vi "fil1_calc.vi"(6 "Detector 3 Correlation In":i32, 7 "Detector 1 Correlation In":i32, 8 "AI1":i32, 9 "AI0":i32) -> (1 "Detector 3 Correlation Out":i32, 3 "Detector 1 Correlation Out":i32)   [LabVIEW 2012]
uses:
  <vilib>/rvi/Emulation/niFpgaSctlEmulationGetInTimedLoop.vi
  <vilib>/rvi/DataTransferAndStorage/Container/Common/niFpgaContainerGetUniqueNameForEmu.vi
  <vilib>/rvi/FIFO/Fifo_Resource/nirvififoEmulationSetSize.vi
  <vilib>/rvi/errors/niFpgaSetErrorForExecOnDevCompSimple.vi
  <vilib>/rvi/eio/common/nirviEmuReportErrorAndStop.vi
  <vilib>/rvi/Emulation/niFpgaSctlEmulationFifoFullMgr.vi
  <vilib>/rvi/Emulation/niFpgaSctlEmulationResourceMgr.vi
  <vilib>/rvi/DataTransferAndStorage/Container/XNode/niFpgaContainer.xnode
  <vilib>/rvi/FIFO/Fifo_Resource/nirvififoEmulationWrite.vi
  <vilib>/rvi/FIFO/Fifo_Resource/nirvififoEmulationRead.vi
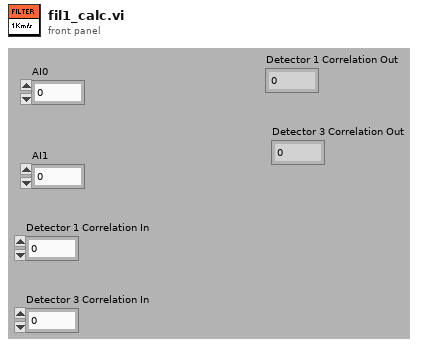
[diagram p1: front panel]
types:
  T1 = cluster{"Average Out":i32, "Next State":u16, "Detector 1 Correlation out":i32, "Detector 3 Correlation out":i32, "Velocity Count out":i32, "Detector counter out":i32, "Timeout count out":u32}
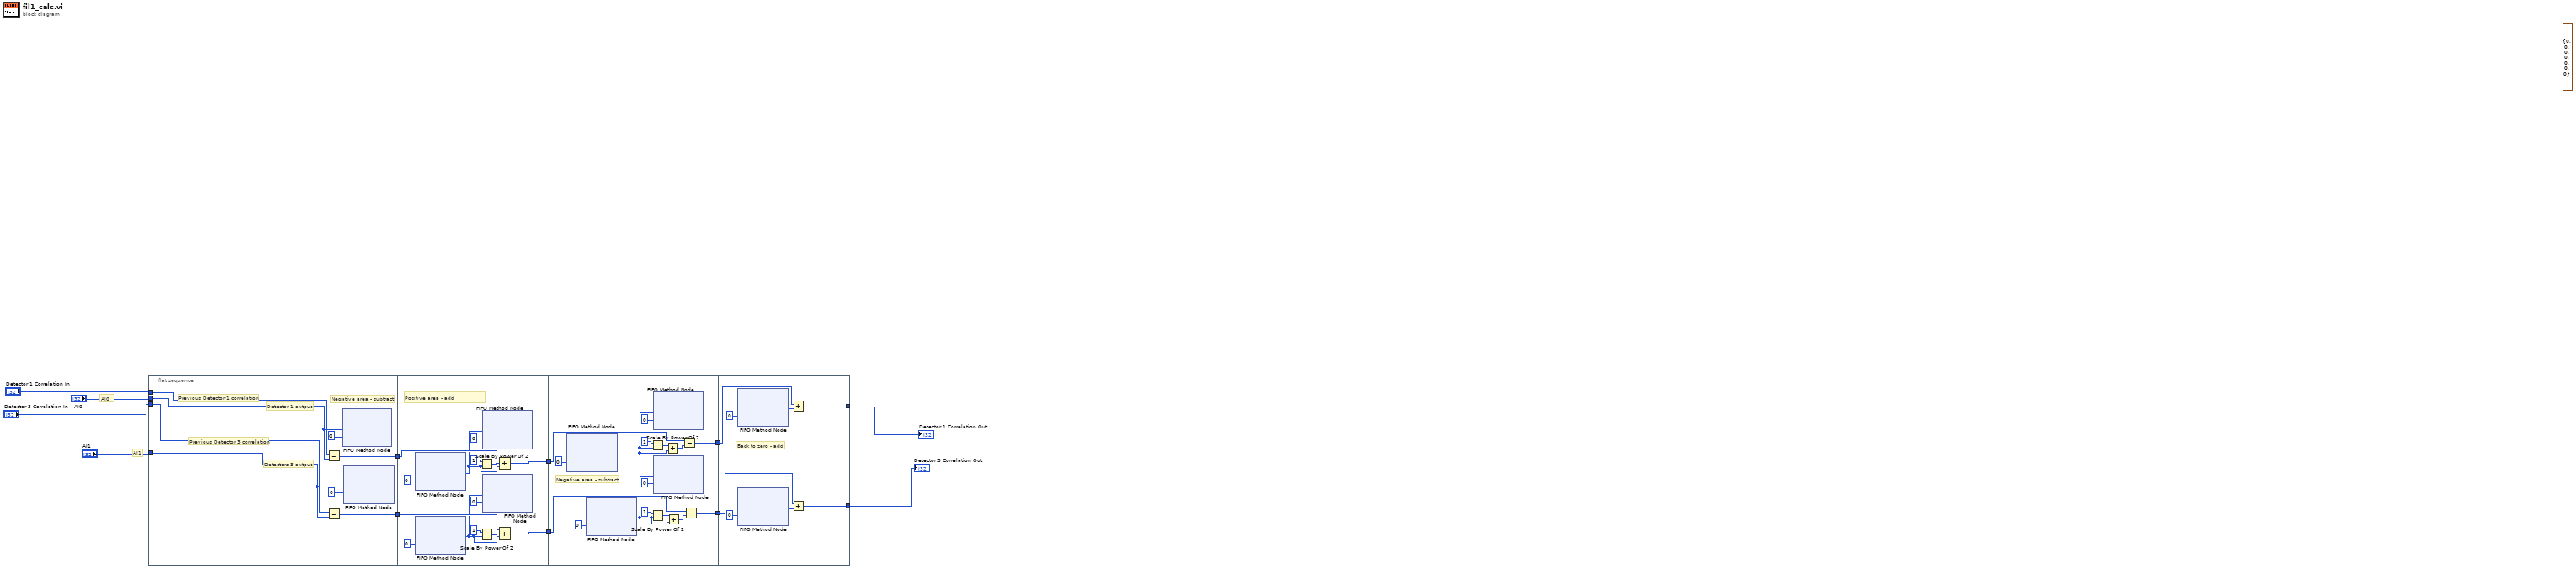
[diagram p0: block diagram]
diagram:
  (unwired) T1 {"Average Out"=0, "Next State"=0, "Detector 1 Correlation out"=0, "Detector 3 Correlation out"=0, "Velocity Count out"=0, "Detector counter out"=0, "Timeout count out"=0} ("Output Cluster")
  # "AI1"
  # "AI0"
  n1 = flat-sequence {
    tunnel: [w19] -> w12
    tunnel: "Detector 1 Correlation In" -> [w18]
    tunnel: "Detector 3 Correlation In" -> [w17]
    tunnel: [w16] -> w11
    tunnel: "AI0" -> [w15]
    tunnel: "AI1" -> [w14]
    tunnel: w12 -> [w33]
    tunnel: [w31] -> w10
    tunnel: w11 -> [w27]
    tunnel: [w25] -> w9
    tunnel: w10 -> [w48]
    tunnel: [w47] -> w8
    tunnel: w9 -> [w42]
    tunnel: [w41] -> w7
    tunnel: w8 -> [w56]
    tunnel: [w55] -> w2
    tunnel: w7 -> [w52]
    tunnel: [w51] -> w1
    frame #0 {
      # "Previous Detector 1 correlation"
      # "Previous Detector 3 correlation"
      # "Detector 1 output"
      # "Detectors 3 output"
      # "Negative area - subtract"
      n2 = Subtract(x=w18, y=w15) -> (x-y=w19:i32)
      n3 = Subtract(x=w17, y=w14) -> (x-y=w16:i32)
      n4 = xnode ("FIFO Method Node")("Element"=w15, "Timeout"=0) -> ()  [unwired: 1 in, 2 out]
      n5 = xnode ("FIFO Method Node")("Element"=w14, "Timeout"=0) -> ()  [unwired: 1 in, 2 out]
    }
    frame #1 {
      # "Positive area - add"
      n6 = xnode ("FIFO Method Node")("Timeout"=0) -> ("Element"=w22:i32)  [unwired: 1 in, 2 out]
      n7 = xnode ("FIFO Method Node")("Timeout"=0) -> ("Element"=w21:i32)  [unwired: 1 in, 2 out]
      n8 = Scale By Power Of 2(n=1, x=w22) -> (x*2^n=w24:i32)
      n9 = Scale By Power Of 2(n=1, x=w21) -> (x*2^n=w23:i32)
      n10 = xnode ("FIFO Method Node")("Element"=w22, "Timeout"=0) -> ()  [unwired: 1 in, 2 out]
      n11 = xnode ("FIFO Method Node")("Element"=w21, "Timeout"=0) -> ()  [unwired: 1 in, 2 out]
      n12 = Compound Arithmetic op=ADD(w33, w24, w22) -> (w31:i32)
      n13 = Compound Arithmetic op=ADD(w27, w23, w21) -> (w25:i32)
    }
    frame #2 {
      # "Negative area - subtract"
      n14 = xnode ("FIFO Method Node")("Timeout"=0) -> ("Element"=w39:i32)  [unwired: 1 in, 2 out]
      n15 = xnode ("FIFO Method Node")("Timeout"=0) -> ("Element"=w36:i32)  [unwired: 1 in, 2 out]
      n16 = Scale By Power Of 2(n=1, x=w39) -> (x*2^n=w40:i32)
      n17 = Scale By Power Of 2(n=1, x=w36) -> (x*2^n=w37:i32)
      n18 = xnode ("FIFO Method Node")("Element"=w39, "Timeout"=0) -> ()  [unwired: 1 in, 2 out]
      n19 = xnode ("FIFO Method Node")("Element"=w36, "Timeout"=0) -> ()  [unwired: 1 in, 2 out]
      n20 = Add(x=w40, y=w39) -> (x+y=w38:i32)
      n21 = Add(x=w37, y=w36) -> (x+y=w35:i32)
      n22 = Subtract(x=w48, y=w38) -> (x-y=w47:i32)
      n23 = Subtract(x=w42, y=w35) -> (x-y=w41:i32)
    }
    frame #3 {
      # "Back to zero - add"
      n24 = xnode ("FIFO Method Node")("Timeout"=0) -> ("Element"=w57:i32)  [unwired: 1 in, 2 out]
      n25 = xnode ("FIFO Method Node")("Timeout"=0) -> ("Element"=w53:i32)  [unwired: 1 in, 2 out]
      n26 = Add(x=w56, y=w57) -> (x+y=w55:i32)
      n27 = Add(x=w52, y=w53) -> (x+y=w51:i32)
    }
  }
  "Detector 1 Correlation Out" <- w2
  "Detector 3 Correlation Out" <- w1
